vi "zup test.vi"() -> ()   [LabVIEW 2014]
uses:
  <vilib>/Instr/_visa.llb/VISA Configure Serial Port (Instr).vi
panel:
  out "read buffer":string
  out "message":string=" INSTRUCTIONS:\r\rNormal Use:  When using subVIs that incorporate the error in/error out (or error I/O) structure, place this handler where you want to inform the user of an error, typically at the end of the I/O data path, as the last action of the program.  If the error in error? is ERROR, the handler creates a message describing the error and its source.  If the type of dialog = 1 (default), the message is displayed to the user, who can only acknowedge it.  If the type = 2, the user can acknowledge the message or abort execution; aborting a program with active I/O is not recommended.  If the type = 0, no message is displayed; this is used to process the error programmatically, and the error out cluster elements are wired to individual terminals for that reason.  \r\rOther Use:\n\r\nlocal testing.  To test the error code of a subVI or function that does not have the error I/O structure, you can wire its error code and a source string to the local error code and error source inputs.  If error in error? indicates no error and error code is not equal to 0, the local code and source are substituted for the error in values, and error? is set TRUE (ERROR)."
  in  "VISA resource name":refnum<visa-resource-name>
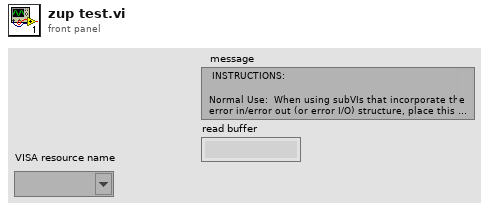
[diagram p1: front panel]
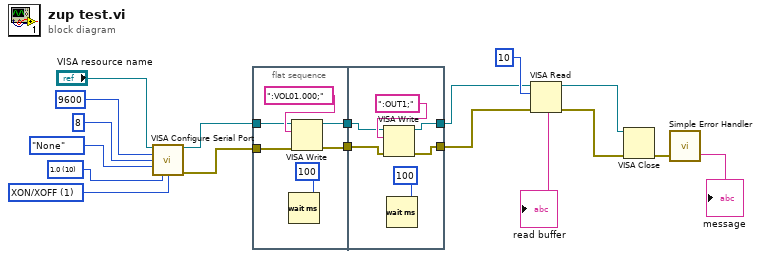
[diagram p0: block diagram]
diagram:
  w18 = u16 1 items=["None", "XON/XOFF", "RTS/CTS", "XON/XOFF & RTS/CTS", "DTR/DSR", "XON/XOFF & DTR/DSR"] ("flow control (0:none)")
  w17 = u16 10 items=["1.0"=10, "1.5"=15, "2.0"=20] ("stop bits (10: 1 bit)")
  n1 = call-poly "VISA Configure Serial Port"("VISA resource name"="VISA resource name", "baud rate (9600)"=u32 9600, "data bits (8)"=u16 8, "parity (0:none)"=enum16{"None", "Odd", "Even", "Mark", "Space"}."None", "stop bits (10: 1 bit)"=w17, "flow control (0:none)"=w18) -> ("VISA resource name out"=w9:refnum<visa-resource-name>, "error out"=w8:errorcluster)  [unwired: 8 in]
  n2 = flat-sequence {
    tunnel: w9 -> [w23]
    tunnel: w8 -> [w22]
    tunnel: [w21] -> w12
    tunnel: [w20] -> w11
    tunnel: [w28] -> w3
    tunnel: [w29] -> w4
    tunnel: w12 -> [w26]
    tunnel: w11 -> [w27]
    frame #0 {
      n3 = Wait (ms)(milliseconds to wait=u32 100) -> ()  [unwired: 1 out]
      n4 = VISA Write(VISA resource name=w23, write buffer=":VOL01.000;", error in (no error)=w22) -> (VISA resource name out=w21:refnum<visa-resource-name>, error out=w20:errorcluster)  [unwired: 1 out]
    }
    frame #1 {
      n5 = VISA Write(VISA resource name=w26, write buffer=":OUT1;", error in (no error)=w27) -> (VISA resource name out=w29:refnum<visa-resource-name>, error out=w28:errorcluster)  [unwired: 1 out]
      n6 = Wait (ms)(milliseconds to wait=u32 100) -> ()  [unwired: 1 out]
    }
  }
  n7 = VISA Read(VISA resource name=w4, byte count=u32 10, error in (no error)=w3) -> (VISA resource name out=w2:refnum<visa-resource-name>, read buffer=→"read buffer":string, error out=w1:errorcluster)  [unwired: 1 out]
  n8 = VISA Close(VISA resource name=w2, error in (no error)=w1) -> (error out=w10:errorcluster)
  n9 = call <vilib>:"Simple Error Handler.vi"("error in (no error)"=w10) -> ("message"=→"message":string)  [unwired: 4 in, 4 out]
